vi "Symbol Modulation (Single Subcarrier).vi"() -> ()   [LabVIEW 2018]
uses:
  <vilib>/Analysis/NI_AALBase.lvlib
  <vilib>/addons/Modulation/niDMT.lvlib
panel:
  out "XY Graph":cluster{"X":dbl, "Y":dbl}[](graph)
  out "Waveform Graph":dbl[](graph)
  out "Constellation Graph":T1(graph)
  in  "QAM":string
  in  "Carrier Freq":dbl
  in  "Symbol \nIn":dbl[](array[numeric])
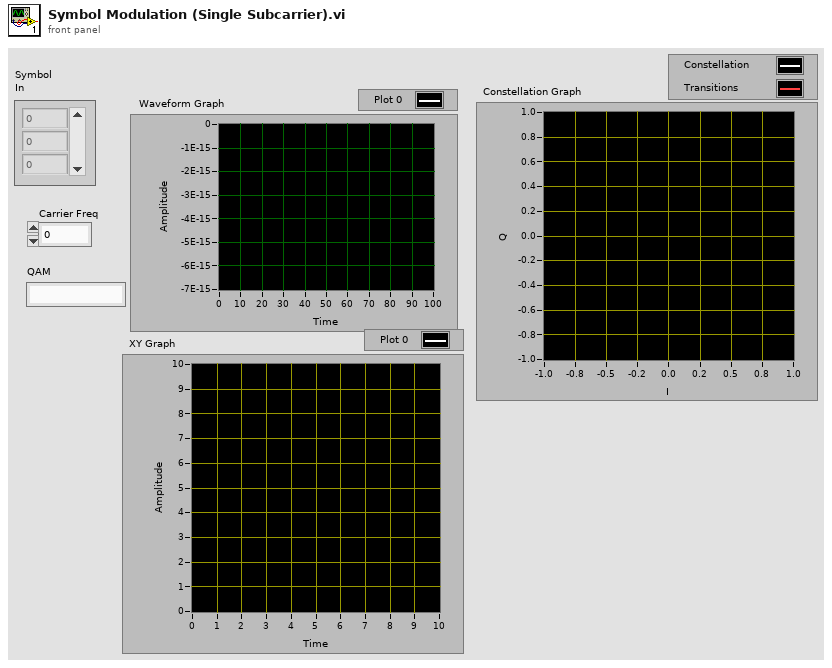
[diagram p1: front panel]
types:
  T1 = cluster{"Decimated Array":dbl[], "Decimated Array":dbl[]}[]
  T2 = cluster{"constellation":dbl[], "oversampled data":dbl[]}[]
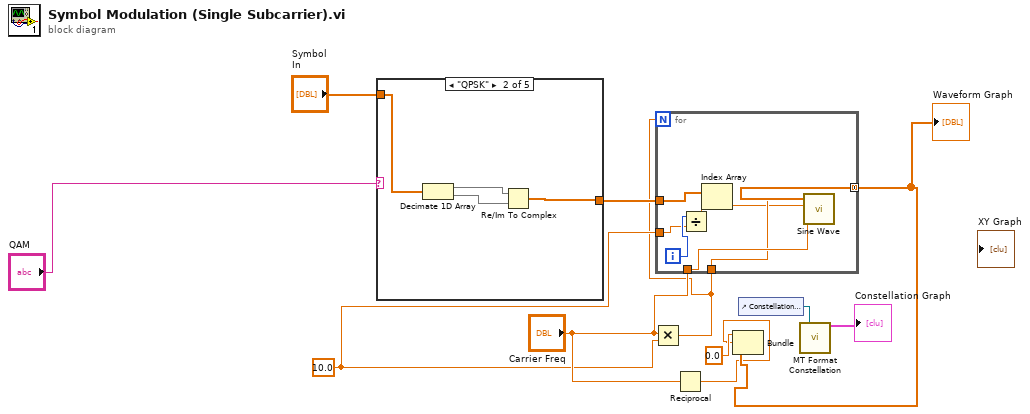
[diagram p0: block diagram]
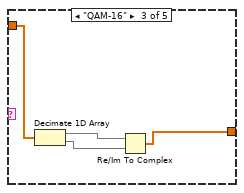
[diagram p3: hidden frame]
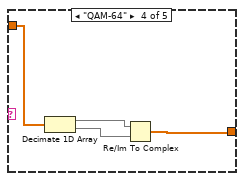
[diagram p4: hidden frame]
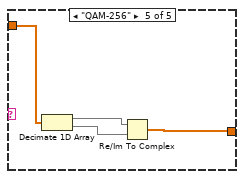
[diagram p5: hidden frame]
diagram:
  w2 = 10.0 ("y")
  n1 = case shown="\"QPSK\"" "QAM" {
    tunnel: "Symbol \nIn" -> [w12 w16 w18 w21 w25]
    tunnel: [w12 w15 w17 w22 w26] -> w9
    frame "BPSK", Default {
    }
    frame "QPSK" {
      n2 = Decimate 1D Array(w16) -> (w14:dbl[], w13:dbl[])
      n3 = Re/Im To Complex(1:w13, 2:w14) -> (0:w15:cdb[])
    }
    frame "QAM-16" {
      n4 = Decimate 1D Array(w18) -> (w20:dbl[], w19:dbl[])
      n5 = Re/Im To Complex(1:w19, 2:w20) -> (0:w17:cdb[])
    }
    frame "QAM-64" {
      n6 = Decimate 1D Array(w21) -> (w24:dbl[], w23:dbl[])
      n7 = Re/Im To Complex(1:w23, 2:w24) -> (0:w22:cdb[])
    }
    frame "QAM-256" {
      n8 = Decimate 1D Array(w25) -> (w28:dbl[], w27:dbl[])
      n9 = Re/Im To Complex(1:w27, 2:w28) -> (0:w26:cdb[])
    }
  }
  n10 = Multiply(x="Carrier Freq", y=w2) -> (x*y=w1:dbl)
  n11 = for {
    N: w1 -> [_]
    tunnel: w9 -> [w33]
    tunnel: [w36] -> w5 mode=concatenating
    tunnel: "Carrier Freq" -> [w35]
    tunnel: w1 -> [w34]
    tunnel: w2 -> [w30]
    i -> [w31]
    n12 = Divide(x=w31, y=w30) -> (x/y=w32:dbl)
    n13 = Index Array(array=w33, index=w32) -> (element=w29:cdb)
    n14 = call <vilib>:"Sine Wave.vi"("samples"=w34, "amplitude"=w29, "frequency"=w35) -> ("sine wave"=w36:dbl[])  [unwired: 2 in, 2 out]
  }
  "Waveform Graph" <- w5
  n15 = Reciprocal(x="Carrier Freq") -> (1/x=w4:dbl)
  n16 = Bundle(0.0, w4, "sine wave"=w5) -> ()  [unwired: 1 in, 1 out]
  n17 = control-ref of="Constellation Graph"() -> (w8:refnum<vi>)
  n18 = call <vilib>:"MT Format Constellation.vi"("constellation reference"=w8) -> ("constellation graph"=→"Constellation Graph":T2)  [unwired: 4 in, 10 out]
